vi "GOMDBTS2048 calib Tristimulus Set XYZ.vi"(7 "valuesZ":dbl[](array[numeric]), 8 "error in (no error)":errorcluster, 9 "valuesY":dbl[](array[numeric]), 10 "valuesX":dbl[](array[numeric]), 11 "handle":i32) -> (0 "error out":errorcluster, 3 "function return":i32)   [LabVIEW 2015, in "GOMDBTS2048.lvlib"]
doc: "GOBTS2048DLL int __stdcall GOMDBTS2048_calibTristimulusSetXYZ(int handle, double* valuesX, double* valuesY, double* valuesZ);"
uses:
  GOMDBTS2048.lvlib
  runtime/GOMDBTS2048.dll
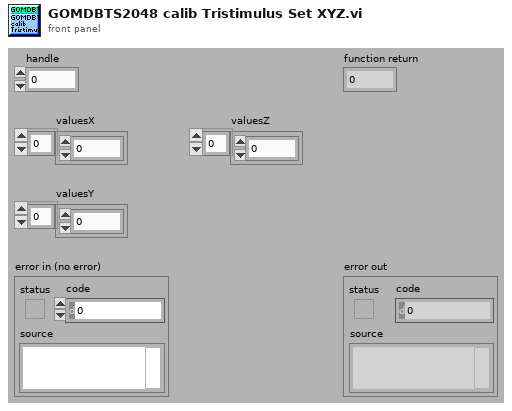
[diagram p1: front panel]
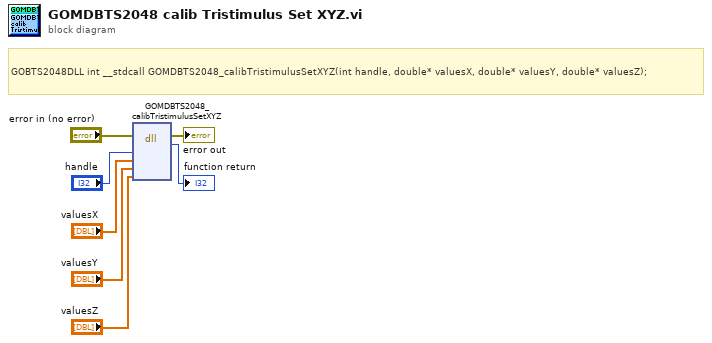
[diagram p0: block diagram]
diagram:
  # "GOBTS2048DLL int __stdcall GOMDBTS2048_calibTristimulusSetXYZ(int handle, double* valuesX, double* valuesY, double* valuesZ);"
  n1 = dll-call lib="C:/Users/rkoch/Documents/GO_Library/runtime/GOMDBTS2048.*" fn="GOMDBTS2048_calibTristimulusSetXYZ"(error in="error in (no error)", "handle"="handle", "valuesX"="valuesX", "valuesY"="valuesY", "valuesZ"="valuesZ") -> (error out=→"error out":errorcluster, →"function return":i32)  [unwired: 6 in, 1 out]
